vi "QI_radial profile.vi"(11 "QI 传递变量输入":T1) -> (1 "radial profile":dbl[](array[numeric]), 2 "array R":dbl[](array[numeric]), 3 "QI 传递变量输出":T1)   [LabVIEW 2017]
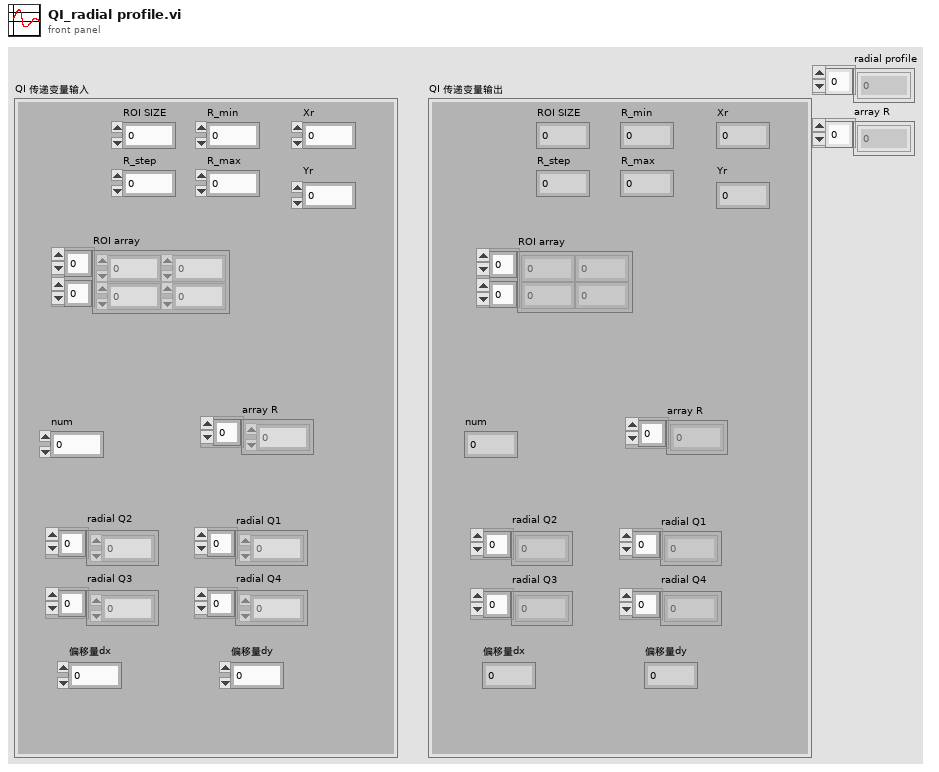
[diagram p1: front panel]
types:
  T1 = typedef "QI 传递变量.ctl" = cluster{"ROI SIZE":i32, "R_step":dbl, "R_min":dbl, "R_max":dbl, "num":dbl, "array R":dbl[], "radial Q1":dbl[], "radial Q2":dbl[], "radial Q3":dbl[], "radial Q4":dbl[], "偏移量dx":dbl, "偏移量dy":dbl, "ROI array":sgl[][], "Xr":dbl, "Yr":dbl}
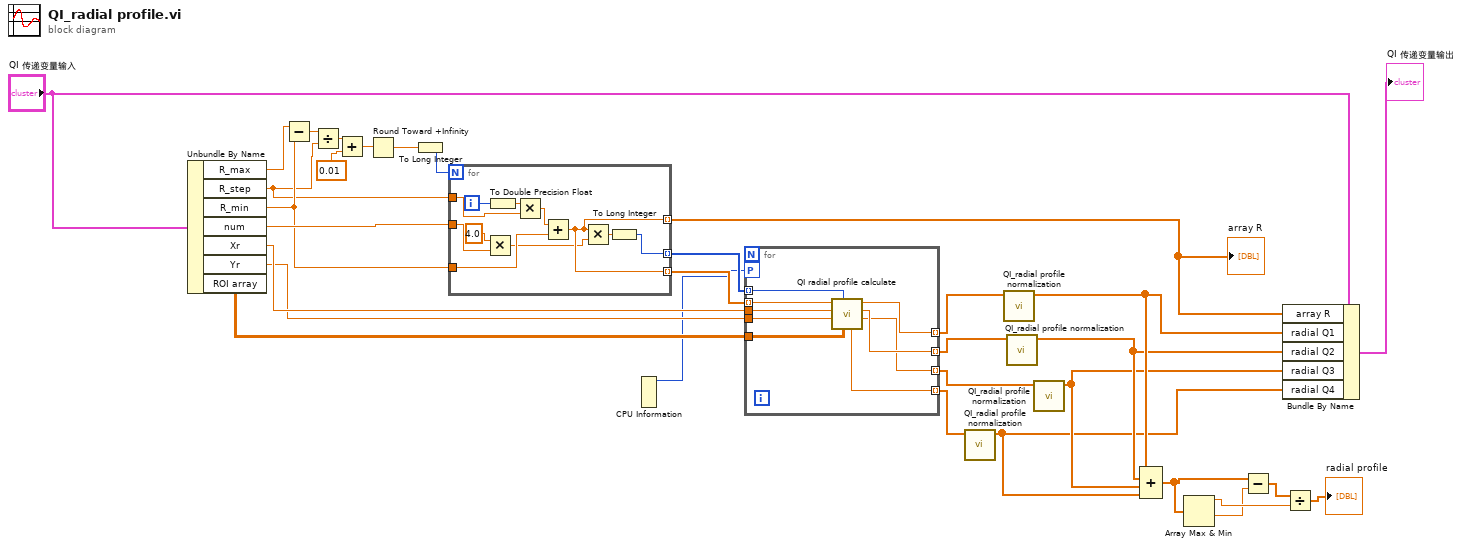
[diagram p0: block diagram]
diagram:
  n1 = Unbundle By Name("QI 传递变量输入") -> ("R_max"=w29:dbl, "R_step"=w26:dbl, "R_min"=w28:dbl, "num"=w30:dbl, "Xr"=w18:dbl, "Yr"=w17:dbl, "ROI array"=w16:sgl[][])
  n2 = Subtract(x=w29, y=w28) -> (x-y=w27:dbl)
  n3 = Divide(x=w27, y=w26) -> (x/y=w25:dbl)
  n4 = Add(x=w25, y=0.01) -> (x+y=w23:dbl)
  n5 = Round Toward +Infinity(x=w23) -> (ceil(x): smallest int >= x=w22:dbl)
  n6 = To Long Integer(number=w22) -> (32bit integer=w21:i32)
  n7 = for "For循环" {
    N: w21 -> [_]
    tunnel: w28 -> [w39]
    tunnel: w26 -> [w41]
    tunnel: w30 -> [w42]
    tunnel: [w35] -> w15 mode=indexing
    tunnel: [w36] -> w20 mode=indexing
    tunnel: [w35] -> w19 mode=indexing
    i -> [w43]
    n8 = Multiply(x=4.0, y=w42) -> (x*y=w34:dbl)
    n9 = To Double Precision Float(number=w43) -> (double precision float=w38:dbl)
    n10 = Multiply(x=w38, y=w41) -> (x*y=w40:dbl)
    n11 = Add(x=w40, y=w39) -> (x+y=w35:dbl)
    n12 = Multiply(x=w35, y=w34) -> (x*y=w37:dbl)
    n13 = To Long Integer(number=w37) -> (32bit integer=w36:i32)
  }
  "array R" <- w15
  n14 = CPU Information() -> (4:w12:i32)  [unwired: 3 out]
  n15 = for "For循环" {
    tunnel: w20 -> [w52] mode=indexing
    tunnel: w19 -> [w51] mode=indexing
    tunnel: w18 -> [w50]
    tunnel: w17 -> [w49]
    tunnel: [w48] -> w5 mode=indexing
    tunnel: [w47] -> w11 mode=indexing
    tunnel: [w46] -> w9 mode=indexing
    tunnel: [w45] -> w7 mode=indexing
    tunnel: w16 -> [w44]
    workers-P: w12 -> [_]
    n16 = call "QI radial profile calculate.vi"("ROI array"=w44, "num"=w52, "Yr"=w49, "Xr"=w50, "r"=w51) -> ("mean3"=w45:dbl, "mean2"=w46:dbl, "mean1"=w47:dbl, "mean4"=w48:dbl)  [unwired: 3 in]
  }
  n17 = call "QI_radial profile normalization.vi"("rp输入"=w5) -> ("rp输出"=w4:dbl[])  [unwired: 10 in]
  n18 = call "QI_radial profile normalization.vi"("rp输入"=w11) -> ("rp输出"=w10:dbl[])  [unwired: 10 in]
  n19 = call "QI_radial profile normalization.vi"("rp输入"=w9) -> ("rp输出"=w8:dbl[])  [unwired: 10 in]
  n20 = call "QI_radial profile normalization.vi"("rp输入"=w7) -> ("rp输出"=w6:dbl[])  [unwired: 10 in]
  n21 = Compound Arithmetic op=ADD(w10, w8, w6, w4) -> (w1:dbl[])
  n22 = Array Max & Min(array=w1) -> (max value=w14:dbl, min value=w2:dbl)  [unwired: 2 out]
  n23 = Subtract(x=w1, y=w2) -> (x-y=w3:dbl[])
  n24 = Bundle By Name(cluster="QI 传递变量输入", "array R"=w15, "radial Q1"=w10, "radial Q2"=w8, "radial Q3"=w6, "radial Q4"=w4) -> (→"QI 传递变量输出":T1)
  n25 = Divide(x=w3, y=w14) -> (x/y=→"radial profile":dbl[])
